vi "Configure Trigger (SetupHold).vi"(0 "VISA resource name":refnum<visa-resource-name>, 1 "Setup Time (1E-9s)":dbl=1e-09, 2 "Hold Time (5E-10s)":dbl=5e-10, 5 "Source":T1={"Data Source (0:Channel1)"=0, "Data Level (1.2V)"=1.2} {"Data Source (0:Channel1)" items=["Channel1", "Channel2", "Channel3", "Channel4"]}, 7 "Clock":T2={"Clock Source (2:Channel2)"=1, "Clock Edge(0:Rise)"=0, "Clock Level (1.2V) "=1.2} {"Clock Edge(0:Rise)" items=["Rise", "Fall"]; "Clock Source (2:Channel2)" items=["Channel1", "Channel2", "Channel3", "Channel4"]}, 11 "error in (no error)":errorcluster, 12 "Trigger If Setup/Hold (0:Occurs)":u16(ring) items=["Occurs", "Logic", "Bus"], 13 "Trigger Event (0:A Event)":u16(ring) items=["A Event", "B Event"]) -> (4 "VISA resource name out":refnum<visa-resource-name>, 6 "Trigger Event Out":u16(ring) items=["A Event", "B Event"], 15 "error out":errorcluster)   [LabVIEW 2011, in "Tektronix 7000 Series.lvlib"]
doc: "Configures sethold trigger settings for an oscilloscope. A setuphold trigger occurs when a setup or hold violation happens.\n\nTDS5000,TDS5000B,TDS6000,CSA7000 and TDS7000 series oscilloscopes don't support B SetupHold Trigger."
uses:
  Tektronix 7000 Series.lvlib
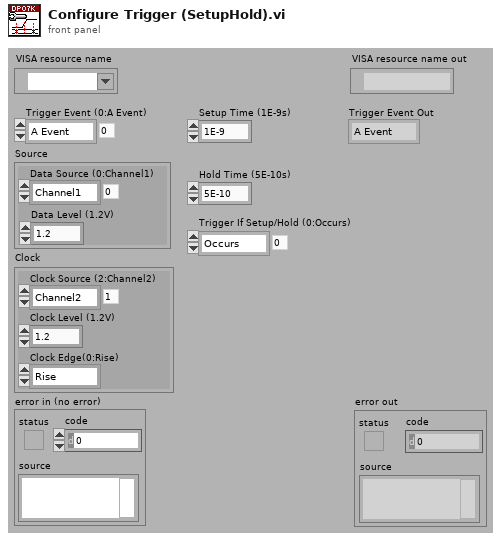
[diagram p1: front panel]
types:
  T1 = cluster{"Data Source (0:Channel1)":u16, "Data Level (1.2V)":dbl}
  T2 = cluster{"Clock Source (2:Channel2)":u16, "Clock Edge(0:Rise)":u16, "Clock Level (1.2V) ":dbl}
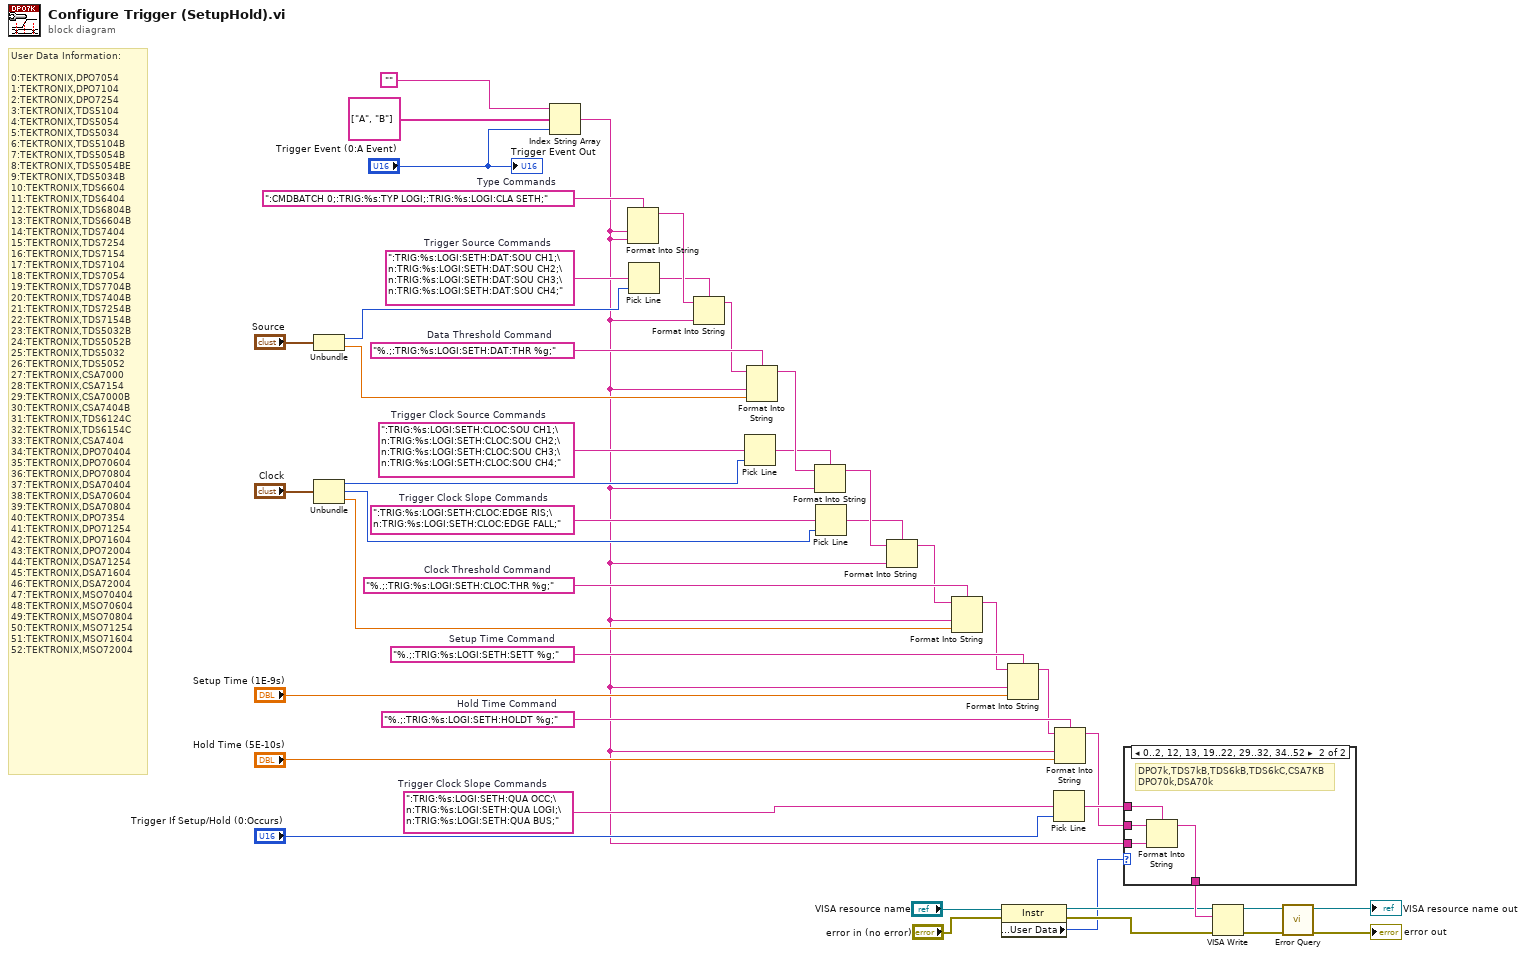
[diagram p0: block diagram]
diagram:
  w26 = "%.;:TRIG:%s:LOGI:SETH:CLOC:THR %g;"  # Clock Threshold Command
  w27 = ":TRIG:%s:LOGI:SETH:QUA OCC;\n:TRIG:%s:LOGI:SETH:QUA LOGI;\n:TRIG:%s:LOGI:SETH:QUA BUS;"  # Trigger Clock Slope Commands
  w28 = ":TRIG:%s:LOGI:SETH:CLOC:EDGE RIS;\n:TRIG:%s:LOGI:SETH:CLOC:EDGE FALL;"  # Trigger Clock Slope Commands
  w29 = ":TRIG:%s:LOGI:SETH:CLOC:SOU CH1;\n:TRIG:%s:LOGI:SETH:CLOC:SOU CH2;\n:TRIG:%s:LOGI:SETH:CLOC:SOU CH3;\n:TRIG:%s:LOGI:SETH:CLOC:SOU CH4;"  # Trigger Clock Source Commands
  w30 = "%.;:TRIG:%s:LOGI:SETH:DAT:THR %g;"  # Data Threshold Command
  w31 = ":TRIG:%s:LOGI:SETH:DAT:SOU CH1;\n:TRIG:%s:LOGI:SETH:DAT:SOU CH2;\n:TRIG:%s:LOGI:SETH:DAT:SOU CH3;\n:TRIG:%s:LOGI:SETH:DAT:SOU CH4;"  # Trigger Source Commands
  w32 = "%.;:TRIG:%s:LOGI:SETH:HOLDT %g;"  # Hold Time Command
  w33 = "%.;:TRIG:%s:LOGI:SETH:SETT %g;"  # Setup Time Command
  w25 = ":CMDBATCH 0;:TRIG:%s:TYP LOGI;:TRIG:%s:LOGI:CLA SETH;"  # Type Commands
  # "User Data Information:\n\n0:TEKTRONIX,DPO7054\n1:TEKTRONIX,DPO7104\n2:TEKTRONIX,DPO7254\n3:TEKTRONIX,TDS5104\n4:TEKTRONIX,TDS5054\n5:TEKTRONIX,TDS5034\n6:TEKTRONIX,TDS5104B\n7:TEKTRONIX,TDS5054B\n8:TEKTRONIX,TDS5054BE\n9:TEKTRONIX,TDS5034B\n10:TEKTRONIX,TDS6604\n11:TEKTRONIX,TDS6404\n12:TEKTRONIX,TDS6804B\n13:TEKTRONIX,TDS6604B\n14:TEKTRONIX,TDS7404\n15:TEKTRONIX,TDS7254\n16:TEKTRONIX,TDS7154\n17:TEKTRONIX,TDS7104\n18:TEKTRONIX,TDS7054\n19:TEKTRONIX,TDS7704B\n20:TEKTRONIX,TDS7404B\n21:TEKTRONIX,TDS7254B\n22:TEKTRONIX,TDS7154B\n23:TEKTRONIX,TDS5032B\n24:TEKTRONIX,TDS5052B\n25:TEKTRONIX,TDS5032\n26:TEKTRONIX,TDS5052\n27:TEKTRONIX,CSA7000\n28:TEKTRONIX,CSA7154\n29:TEKTRONIX,CSA7000B\n30:TEKTRONIX,CSA7404B\n31:TEKTRONIX,TDS6124C\n32:TEKTRONIX,TDS6154C\n33:TEKTRONIX,CSA7404\n34:TEKTRONIX,DPO70404\n35:TEKTRONIX,DPO70604\n36:TEKTRONIX,DPO70804\n37:TEKTRONIX,DSA70404\n38:TEKTRONIX,DSA70604\n39:TEKTRONIX,DSA70804\n40:TEKTRONIX,DPO7354\n41:TEKTRONIX,DPO71254\n42:TEKTRONIX,DPO71604\n43:TEKTRONIX,DPO72004\n44:TEKTRONIX,DSA71254\n45:TEKTRONIX,DSA71604\n46:TEKTRONIX,DSA72004\n47:TEKTRONIX,MSO70404\n48:TEKTRONIX,MSO70604\n49:TEKTRONIX,MSO70804\n50:TEKTRONIX,MSO71254\n51:TEKTRONIX,MSO71604\n52:TEKTRONIX,MSO72004"
  n1 = Unbundle("Source") -> ("Data Source (0:Channel1)"=w24:u16, "Data Level (1.2V)"=w20:dbl)
  n2 = Unbundle("Clock") -> ("Clock Source (2:Channel2)"=w43:u16, "Clock Edge(0:Rise)"=w42:u16, "Clock Level (1.2V)"=w14:dbl)
  n3 = Index String Array(1:"Trigger Event (0:A Event)", 2:string[] ["A", "B"], 3:"" ("Empty String Constant")) -> (0:w8:string)
  n4 = Format Into String(format string=w25, w8, w8) -> (resulting string=w23:string)  [unwired: 2 in, 1 out]
  n5 = Pick Line(multi-line string=w31, line index=w24) -> (output string=w22:string)  [unwired: 1 in]
  n6 = Format Into String(format string=w22, initial string=w23, w8) -> (resulting string=w21:string)  [unwired: 1 in, 1 out]
  n7 = Pick Line(multi-line string=w29, line index=w43) -> (output string=w18:string)  [unwired: 1 in]
  n8 = Format Into String(format string=w30, initial string=w21, w8, w20) -> (resulting string=w19:string)  [unwired: 1 in, 1 out]
  n9 = Format Into String(format string=w18, initial string=w19, w8) -> (resulting string=w17:string)  [unwired: 1 in, 1 out]
  n10 = Pick Line(multi-line string=w28, line index=w42) -> (output string=w16:string)  [unwired: 1 in]
  n11 = Format Into String(format string=w16, initial string=w17, w8) -> (resulting string=w15:string)  [unwired: 1 in, 1 out]
  n12 = Format Into String(format string=w26, initial string=w15, w8, w14) -> (resulting string=w12:string)  [unwired: 1 in, 1 out]
  n13 = property class="Instr"(reference="VISA resource name", error in="error in (no error)") -> (reference out=w4:refnum<visa-resource-name>, error out=w3:errorcluster, "General Settings:User Data"=w1:u32)
  n14 = Format Into String(format string=w33, initial string=w12, w8, "Setup Time (1E-9s)") -> (resulting string=w11:string)  [unwired: 1 in, 1 out]
  n15 = Pick Line(multi-line string=w27, line index="Trigger If Setup/Hold (0:Occurs)") -> (output string=w9:string)  [unwired: 1 in]
  n16 = Format Into String(format string=w32, initial string=w11, w8, "Hold Time (5E-10s)") -> (resulting string=w2:string)  [unwired: 1 in, 1 out]
  n17 = case shown="0..2, 12, 13, 19..22, 29..32, 34..52" w1 {
    tunnel: w9 -> [_ w50]
    tunnel: w8 -> [_ w49]
    tunnel: [w46 w48] -> w7
    tunnel: w2 -> [w46 w47]
    frame Default {
    }
    frame 0..2, 12, 13, 19..22, 29..32, 34..52 {
      # "DPO7k,TDS7kB,TDS6kB,TDS6kC,CSA7KB\nDPO70k,DSA70k"
      n18 = Format Into String(format string=w50, initial string=w47, w49) -> (resulting string=w48:string)  [unwired: 1 in, 1 out]
    }
  }
  n19 = VISA Write(VISA resource name=w4, write buffer=w7, error in (no error)=w3) -> (VISA resource name out=w39:refnum<visa-resource-name>, error out=w40:errorcluster)  [unwired: 1 out]
  n20 = call "Error Query.vi"("error in (no error)"=w40, "VISA resource name"=w39) -> ("error out"=→"error out":errorcluster, "VISA resource name out"=→"VISA resource name out":refnum<visa-resource-name>)  [unwired: 6 in, 2 out]
  "Trigger Event Out" <- "Trigger Event (0:A Event)"
